vi "CheckSystemSettingControl.vi"(8 "error in (no error)":errorcluster, 11 "SR430Class in":refnum<class "SR430Class.lvclass">) -> (0 "error out":errorcluster, 2 "Enable/Disable Controls":string, 3 "SR430Class out":refnum<class "SR430Class.lvclass">)   [LabVIEW 2015, in "SR430Class.lvclass"]
uses:
  class/SR430Class.lvclass
  class/SR430Class.lvclass/SR430Class.ctl
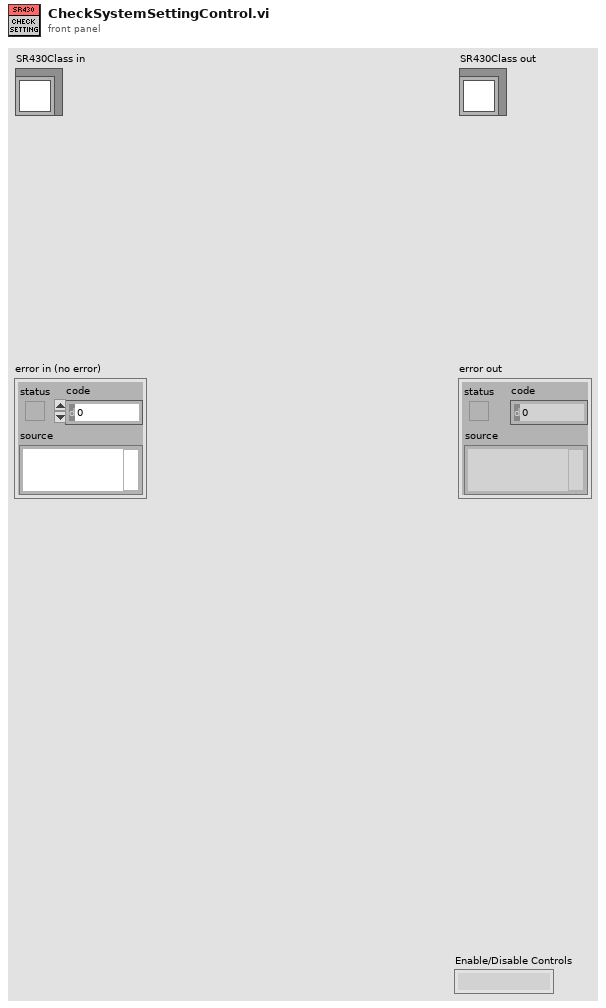
[diagram p1: front panel]
types:
  T1 = enum8{"Enabled", "Disabled", "Disabled and Grayed Out"}
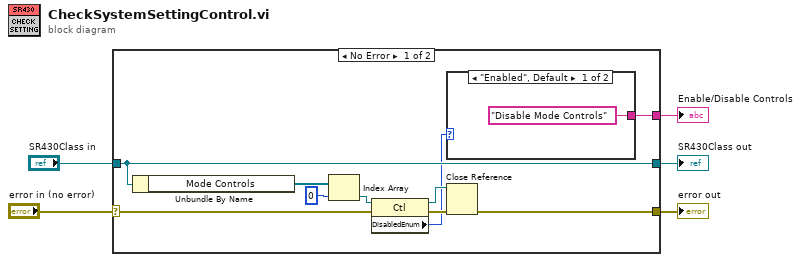
[diagram p0: block diagram]
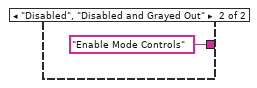
[diagram p2: hidden frame]
diagram:
  n1 = case shown="No Error" "error in (no error)" {
    selector: "error in (no error)" -> [w11 w19]
    tunnel: [w9 w19] -> w2
    tunnel: [w15 w18] -> w3
    tunnel: "SR430Class in" -> [w15 w18]
    tunnel: [w6 _] -> w5
    frame No Error {
      n2 = Unbundle By Name(w15) -> ("Mode Controls"=w14:refnum<vi>[])
      n3 = Index Array(array=w14, index=0) -> (element=w12:refnum<vi>)
      n4 = property class="Ctl"(reference=w12, error in=w11) -> (reference out=w10:refnum<vi>, error out=w8:errorcluster, "DisabledEnum"=w7:T1)
      n5 = case shown="\"Enabled\", Default" w7 {
        tunnel: ["Disable Mode Controls" "Enable Mode Controls"] -> w6
        frame "Enabled", Default {
        }
        frame "Disabled", "Disabled and Grayed Out" {
        }
      }
      n6 = Close Reference(reference=w10, error in (no error)=w8) -> (error out=w9:errorcluster)
    }
    frame Error {
    }
  }
  "error out" <- w2
  "SR430Class out" <- w3
  "Enable/Disable Controls" <- w5
